vi "Add Time Stamp.vi"(8 "error in (no error)":errorcluster, 11 "Loopback in":refnum<class "Loopback.lvclass">) -> (0 "error out":errorcluster, 3 "Loopback out":refnum<class "Loopback.lvclass">)   [LabVIEW 2014, in "Loopback.lvclass"]
uses:
  Loopback.lvclass
  Loopback.lvclass/Loopback.ctl
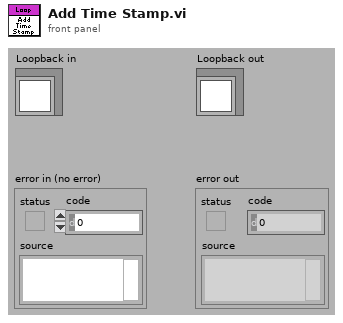
[diagram p1: front panel]
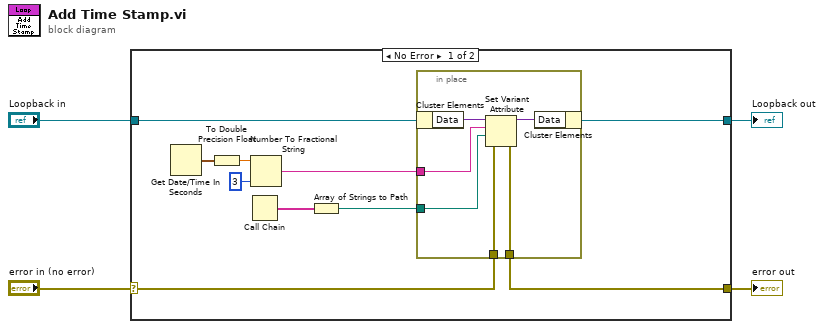
[diagram p0: block diagram]
diagram:
  n1 = case shown="No Error" "error in (no error)" {
    selector: "error in (no error)" -> [w7 w22]
    tunnel: [w6 w22] -> w3
    tunnel: [w13 w21] -> w1
    tunnel: "Loopback in" -> [w14 w21]
    frame No Error {
      n2 = Get Date/Time In Seconds() -> (seconds since 1Jan1904=w10:timestamp)
      n3 = To Double Precision Float(number=w10) -> (double precision float=w11:dbl)
      n4 = Call Chain() -> (call chain=w8:string[])
      n5 = Number To Fractional String(number=w11, precision (6)=i16 3) -> (F-format string=w9:string)  [unwired: 2 in]
      n6 = Array of Strings to Path(0:w8) -> (2:w5:path)  [unwired: 1 in]
      n7 = in-place {
        in-place-border: w9 -> [w18]
        in-place-border: w5 -> [w17]
        in-place-border: w7 -> [w16]
        in-place-border: [w15] -> w6
        n8 = in-place-cluster #1(w14) -> ("Data"=w20:variant)
        n9 = Set Variant Attribute(Variant=w20, name=w18, value=w17, error in=w16) -> (Variant out=w19:variant, error out=w15:errorcluster)  [unwired: 1 out]
        n10 = in-place-cluster #1("Data"=w19) -> (w13:refnum<class "Loopback.lvclass">)
      }
    }
    frame Error {
    }
  }
  "error out" <- w3
  "Loopback out" <- w1
